vi "WhiteNoiseGlobal.vi"() -> ()   [LabVIEW 2012]
panel:
  in  "Cutoff (Hz)":dbl=1000.0 format="%0.2f"
  in  "amplitude":dbl=1.0 format="%.2p"
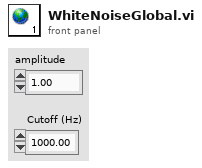
[diagram p1: front panel]
diagram:
